vi "Generate SysDef Path.vi"() -> (0 "System Definition path":path)   [LabVIEW 2019, in "Scalar Bitpacking Testing.lvclass"]
uses:
  Scalar Bitpacking Testing.lvclass
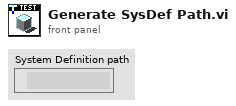
[diagram p1: front panel]
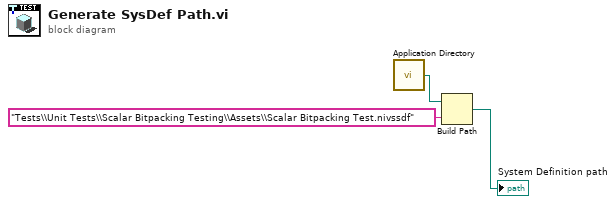
[diagram p0: block diagram]
diagram:
  n1 = call <vilib>:"Application Directory.vi"() -> ("Application Directory"=w1:path)
  n2 = Build Path(base path=w1, name or relative path="Tests\\Unit Tests\\Scalar Bitpacking Testing\\Assets\\Scalar Bitpacking Test.nivssdf") -> (appended path=→"System Definition path":path)
